vi "Analogue 1 Direct.vi"(2 "Vps 6":fxp<+/-,20,5> format="%.17g", 3 "Vps 5":fxp<+/-,20,5> format="%.17g", 8 "Vps 4":fxp<+/-,20,5> format="%.17g", 9 "Vps 3":fxp<+/-,20,5> format="%.17g", 10 "Vps 2":fxp<+/-,20,5> format="%.17g", 11 "Vps 1":fxp<+/-,20,5> format="%.17g") -> ()   [LabVIEW 2023]
uses:
  <vilib>/rvi/Emulation/niFpgaGetClockAttributes.vi
  <vilib>/rvi/Emulation/niFpgaSctlEmulationGetInTimedLoop.vi
  <vilib>/rvi/Emulation/niFpgaEmulationReportErrorSimple.vi
  <vilib>/rvi/eio/common/nirviEmuTemplateMethod_errors.vi
  <vilib>/rvi/Emulation/niFpgaCriticalErrorInLSC.vi
  <vilib>/eio/EIONode/EIONode.xnode
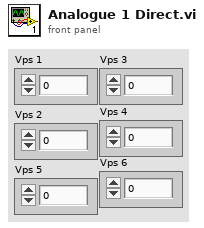
[diagram p1: front panel]
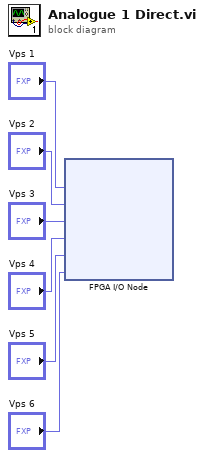
[diagram p0: block diagram]
diagram:
  n1 = xnode "FPGA I/O Node"("Mod8/AO0"="Vps 1", "Mod8/AO2"="Vps 2", "Mod8/AO4"="Vps 3", "Mod8/AO6"="Vps 4", "Mod8/AO8"="Vps 5", "Mod8/AO10"="Vps 6") -> ()  [unwired: 6 in, 6 out]
